vi "APPA207.vi"(4 "error in":T13, 7 "Command":T14) -> (0 "error out":T13, 3 "Response":T11)   [LabVIEW 2018]
uses:
  MOKO_LabViewLibrary/MokoLowLevel/MokoLowLovelControl/MLLC_Command.ctl
  MOKO_LabViewLibrary/MokoLowLevel/MokoLowLovelControl/MLLC_Error.ctl
  MOKO_LabViewLibrary/MokoLowLevel/MokoLowLovelControl/MLLC_Mode.ctl
  MOKO_LabViewLibrary/MokoLowLevel/MokoLowLovelControl/MLLC_Response.ctl
  MOKO_LabViewLibrary/MokoLowLevel/MokoLowLovelControl/MLLC_DriverName.ctl
  MOKO_LabViewLibrary/MokoLowLevel/MokoLowLovelControl/MLLC_Request.ctl
  MOKO_LabViewLibrary/MokoLowLevel/MokoLowLovelControl/MLLC_ErrorCode.ctl
  MOKO_LabViewLibrary/MokoLowLevel/MokoLowLovelControl/MLLC_ConnectCluster.ctl
  MOKO_LabViewLibrary/MokoLowLevel/MokoLowLovelControl/MLLC_InterfaceType.ctl
  MOKO_LabViewLibrary/MokoLowLevel/MokoLowLovelControl/MLLC_OpenedSession.ctl
  MOKO_LabViewLibrary/MokoLowLevel/MokoLowLovelControl/MLLC_InterfaceSettings.ctl
  MOKO_LabViewLibrary/MokoLowLevel/MokoLowLovelControl/MLLC_InterfaceKind.ctl
  MOKO_LabViewLibrary/MokoLowLevel/MokoLowLovelControl/MLLC_ResponseInit.ctl
  MOKO_LabViewLibrary/MokoLowLevel/MokoLowLovelControl/MLLC_Rs232Settings.ctl
panel:
  in  "ResponseInit":T1="OK"
  in  "Settings":T7={"Permanent data"={"Connect"={"InterfaceType"=enum."VISA", "OpenedSession"="", "InterfaceSettings"={"Interface"=enum."RS232", "EOS 4 read"=enum."None", "EOS 4 write"=enum."None", "TMO, ms"=1000, "Sett"=variant(cluster{"Baud Rate":u32, "Data Bits":u16, "Parity":u16, "Stop Bits":u16, "Flow Control":u16, "Eho":bool} {"Baud Rate"=75, "Data Bits"=0, "Parity"=0, "Stop Bits"=0, "Flow Control"=0, "Eho"=FALSE})}}}, "Saved Data"=variant}
  in  "Error Code":T8=5475
  in  "Request":T9="UU\u0000\u0000ª"
  in  "Driver Name":T10="APPA207"
  in  "Mode":T12=enum."Check"
  # "APPA207"
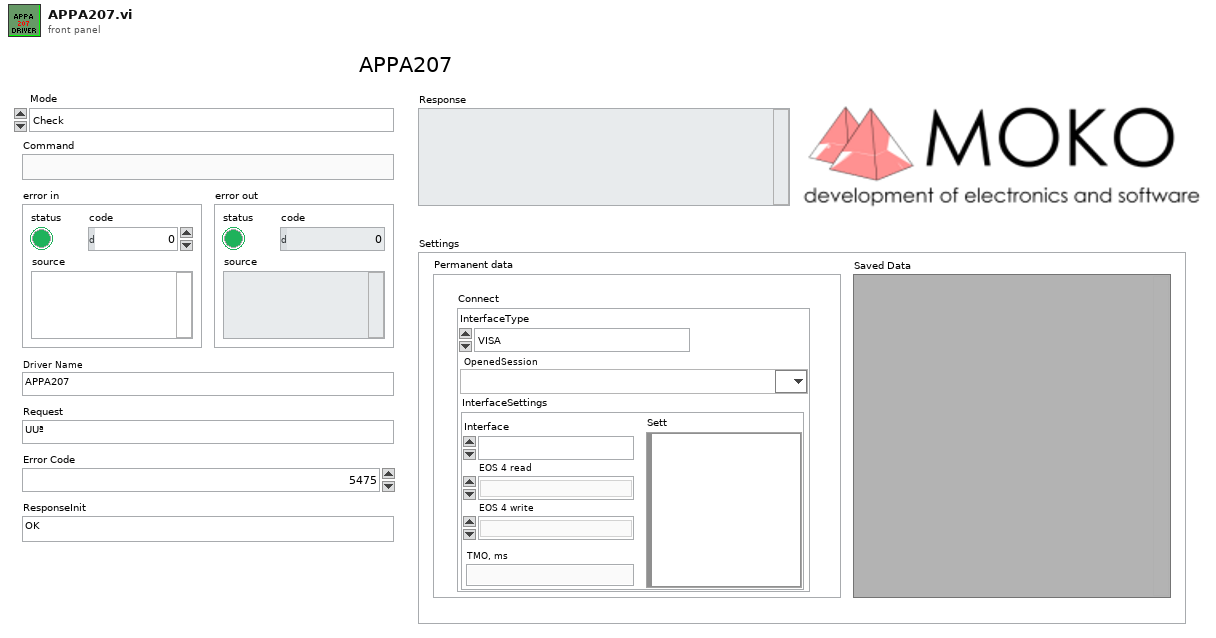
[diagram p1: front panel]
types:
  T1 = typedef "MLLC_ResponseInit.ctl" = string
  T2 = typedef "MLLC_ConnectCluster.ctl" = cluster{"InterfaceType":T3, "OpenedSession":T4, "InterfaceSettings":T5}
  T3 = typedef "MLLC_InterfaceType.ctl" = enum16{"VISA", "Prologix USB-GPIB"}
  T4 = typedef "MLLC_OpenedSession.ctl" = refnum<visa-resource-name>
  T5 = typedef "MLLC_InterfaceSettings.ctl" = cluster{"Interface":T6, "EOS 4 read":enum16{"Default (=EOS 4 write)", "CR (\\r)", "LF (\\n)", "None"}, "EOS 4 write":enum16{"CR+LF (\\r\\n)", "CR (\\r)", "LF (\\n)", "None"}, "TMO, ms":i32, "Sett":variant}
  T6 = typedef "MLLC_InterfaceKind.ctl" = enum16{"RS232", "GPIB", "USB", "Ethernet", "another"}
  T7 = cluster{"Permanent data":cluster{"Connect":T2}, "Saved Data":variant}
  T8 = typedef "MLLC_ErrorCode.ctl" = u32
  T9 = typedef "MLLC_Request.ctl" = string
  T10 = typedef "MLLC_DriverName.ctl" = string
  T11 = typedef "MLLC_Response.ctl" = string
  T12 = typedef "MLLC_Mode.ctl" = enum16{"get", "set", "close", "Init", "Check"}
  T13 = typedef "MLLC_Error.ctl" = errorcluster
  T14 = typedef "MLLC_Command.ctl" = string
  T15 = typedef "MLLC_Rs232Settings.ctl" = cluster{"Baud Rate":u32, "Data Bits":u16, "Parity":u16, "Stop Bits":u16, "Flow Control":u16, "Eho":bool, "Address":dbl}
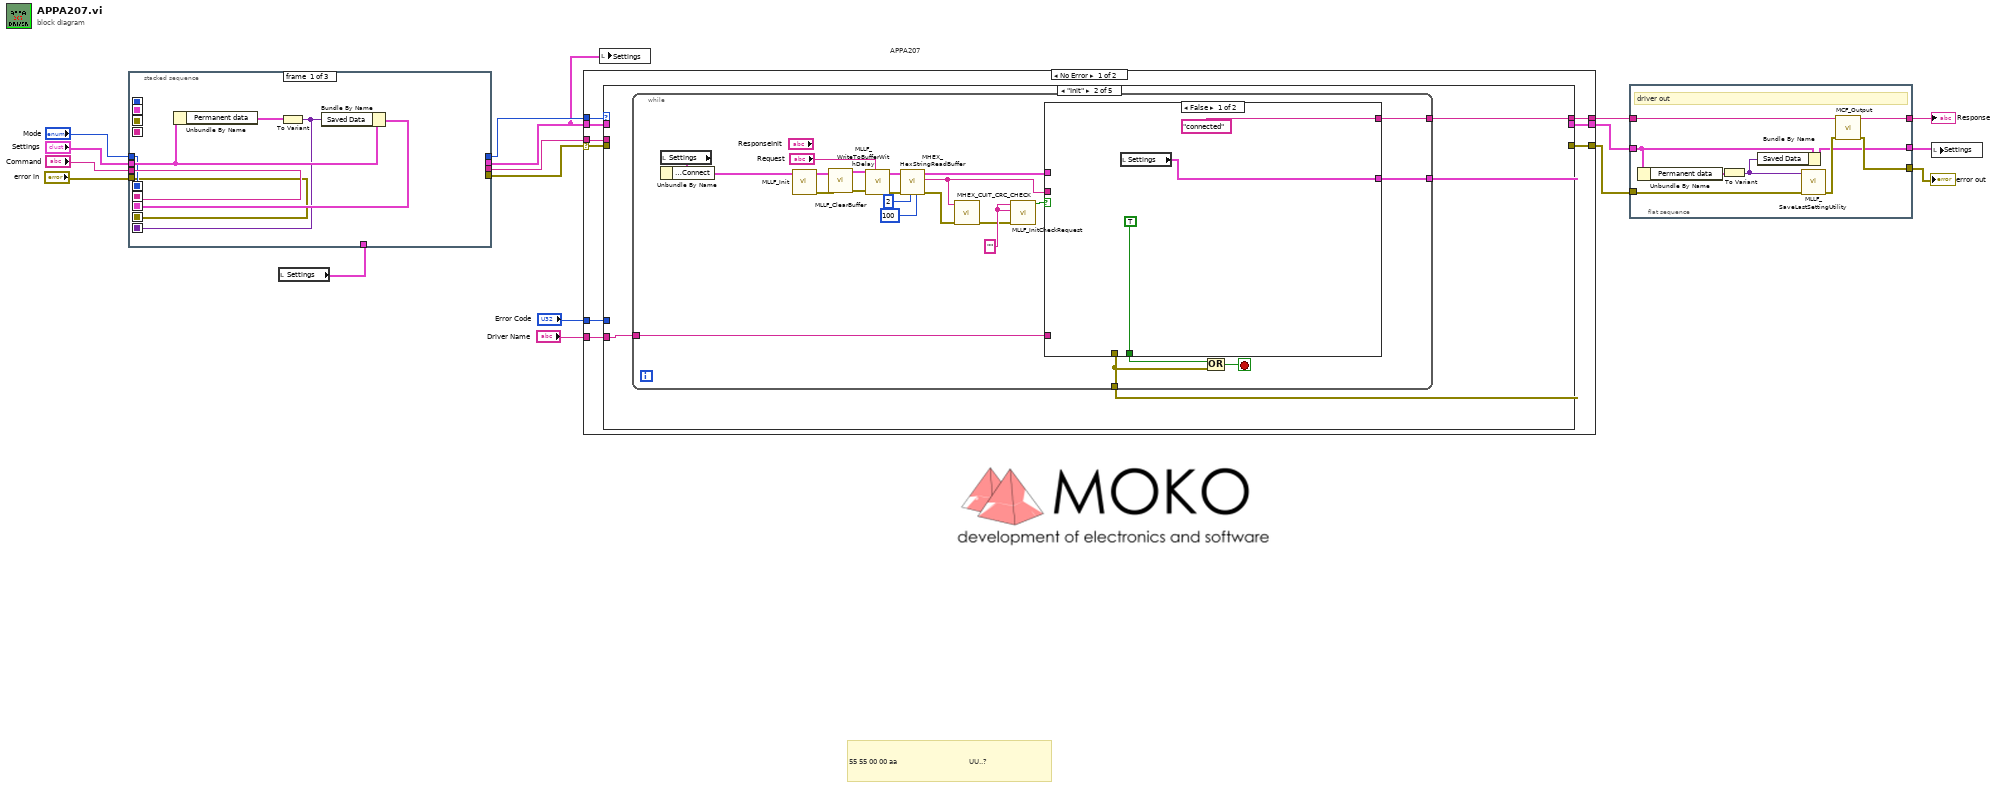
[diagram p0: block diagram]
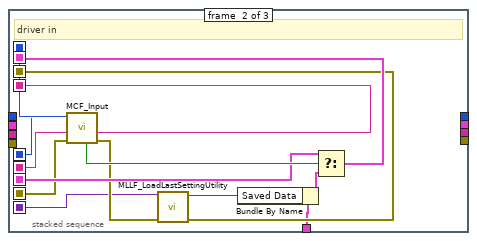
[diagram p2: hidden frame]
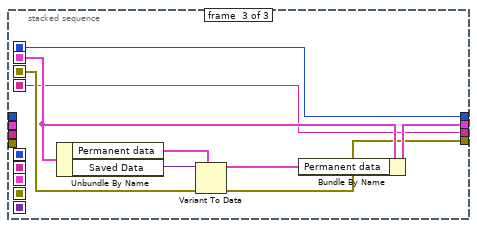
[diagram p3: hidden frame]
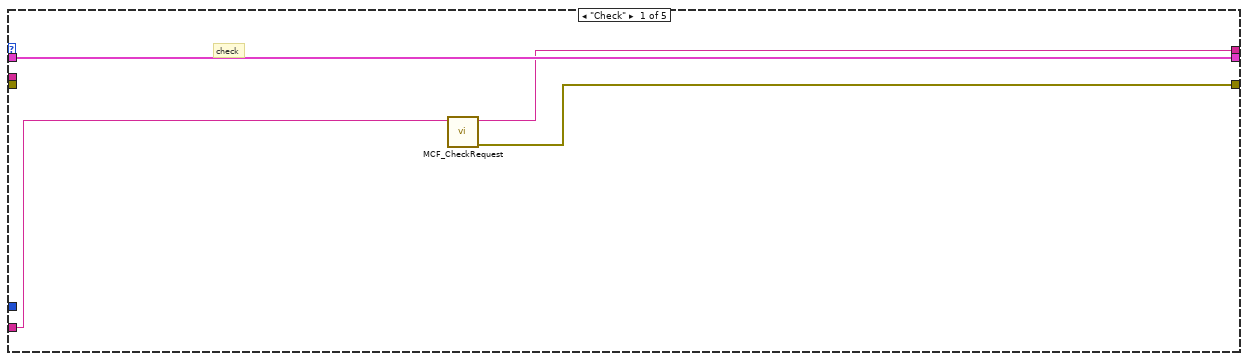
[diagram p4: hidden frame]
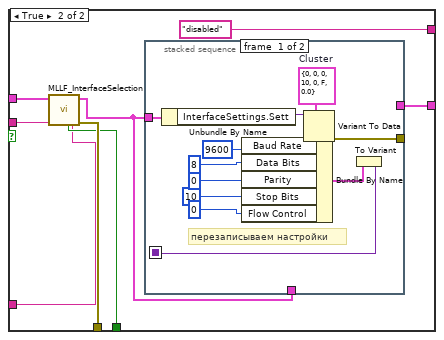
[diagram p5: hidden frame]
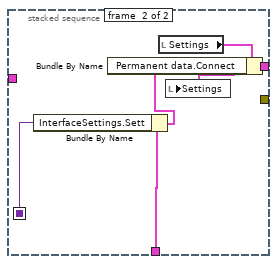
[diagram p6: hidden frame]
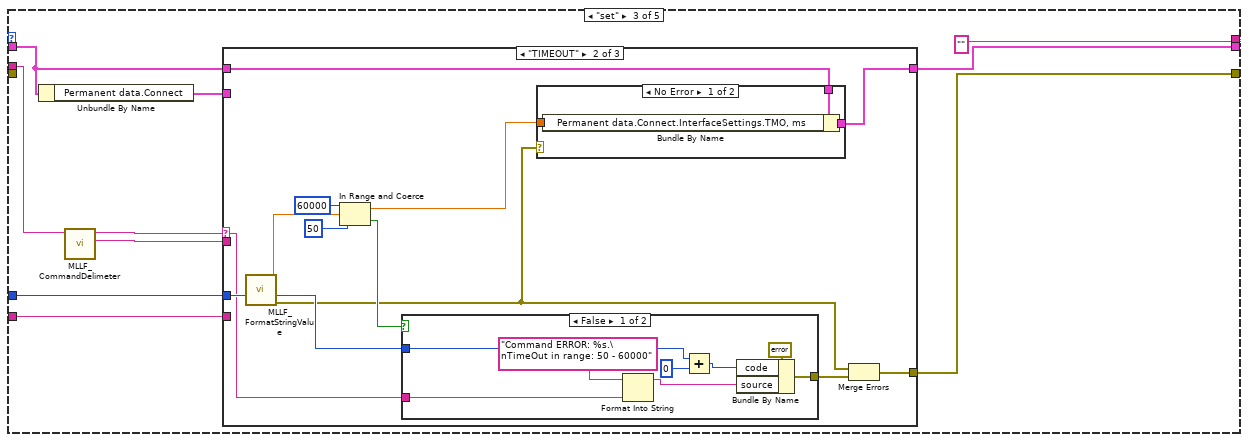
[diagram p7: hidden frame]
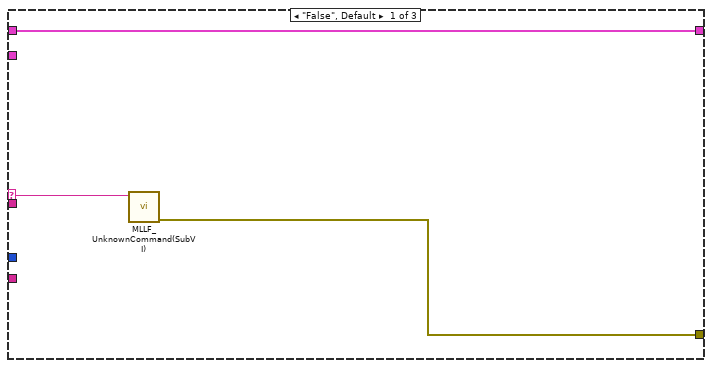
[diagram p8: hidden frame]
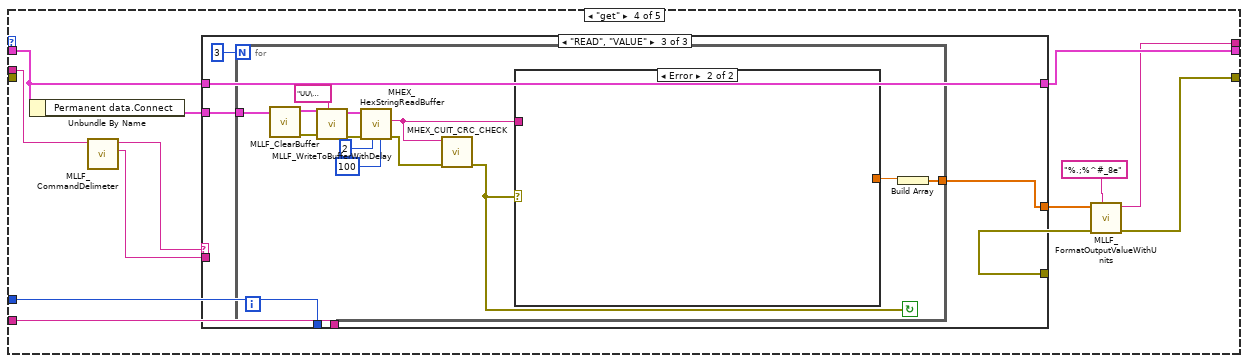
[diagram p12: hidden frame]
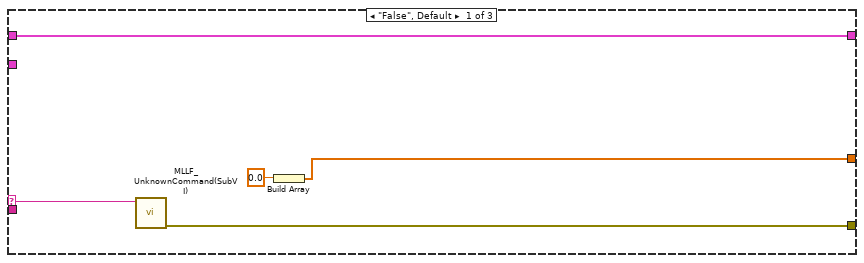
[diagram p13: hidden frame]
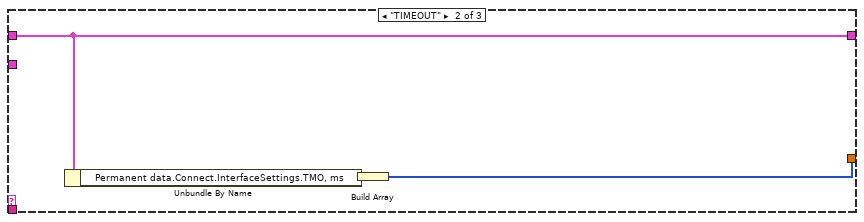
[diagram p14: hidden frame]
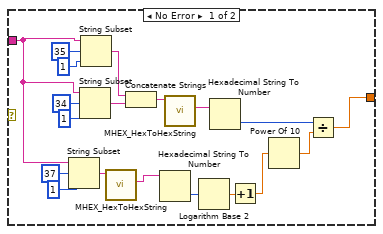
[diagram p15: hidden frame]
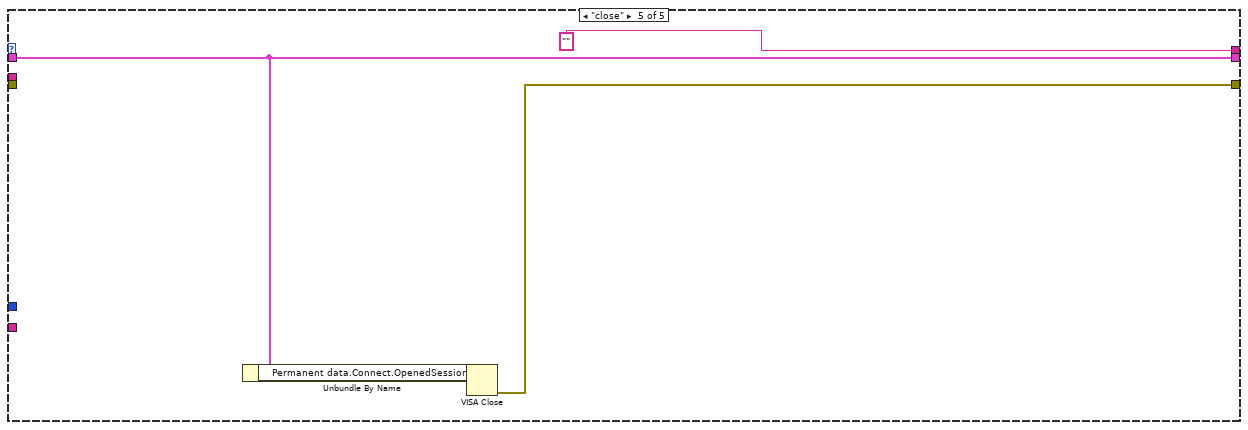
[diagram p16: hidden frame]
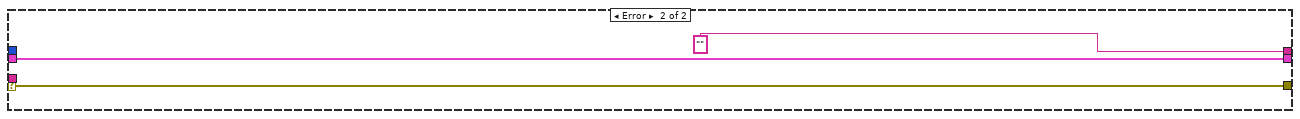
[diagram p17: hidden frame]
diagram:
  # "55 55 00 00 aa                                    UU..?"
  # "APPA207"
  n1 = local read "Settings"() -> (w11:T7)
  n2 = stacked-sequence {
    seq-local: [w20 _ _] -> [_ w36 _]
    seq-local: [w19 _ _] -> [_ w37 _]
    seq-local: [w22 _ _] -> [_ w32 _]
    seq-local: [w18 _ _] -> [_ w31 _]
    seq-local: [w21 _ _] -> [_ w27 _]
    seq-local: [_ w28 _] -> [_ _ w44]
    seq-local: [_ w38 _] -> [_ _ w41]
    seq-local: [_ w35 _] -> [_ _ w40]
    seq-local: [_ w34 _] -> [_ _ w45]
    tunnel: "Command" -> [w20 _ _]
    tunnel: "Mode" -> [w19 _ _]
    tunnel: "error in" -> [w18 _ _]
    tunnel: "Settings" -> [w23 _ _]
    tunnel: w11 -> [_ w26 _]
    tunnel: [_ _ w40] -> w8
    tunnel: [_ _ w43] -> w9
    tunnel: [_ _ w42] -> w7
    tunnel: [_ _ w41] -> w10
    frame #0 {
      n3 = Unbundle By Name(w23) -> ("Permanent data"=w24:cluster{"Connect":T2})
      n4 = To Variant(anything=w24) -> (Variant=w21:variant)
      n5 = Bundle By Name(cluster=w23, "Saved Data"=w21) -> (w22:T7)
    }
    frame #1 {
      # "driver in"
      n6 = call "MCF_Input.vi"("Error In"=w31, "Command in"=w36, "Mode in"=w37) -> ("Error Out"=w30:errorcluster, "Command out"=w35:string, "Mode out"=w38:T12, "Boolean"=w33:bool)  [unwired: 5 in]
      n7 = call "MLLF_LoadLastSettingUtility.vi"("Error In"=w30, "Save data in"=w27) -> ("Error Out"=w28:errorcluster, "Save data out"=w25:variant)  [unwired: 8 in]
      n8 = Bundle By Name(cluster=w26, "Saved Data"=w25) -> (w29:T7)
      n9 = Select(t=w32, s=w33, f=w29) -> (s? t:f=w34:T7)
    }
    frame #2 {
      n10 = Unbundle By Name(w45) -> ("Permanent data"=w46:cluster{"Connect":T2}, "Saved Data"=w39:variant)
      n11 = Variant To Data(error in=w44, type=w46, Variant=w39) -> (data=w47:cluster{"Connect":T2}, error out=w42:errorcluster)
      n12 = Bundle By Name(cluster=w45, "Permanent data"=w47) -> (w43:T7)
    }
  }
  n13 = case shown="No Error" w7 {
    selector: w7 -> [w52 w217]
    tunnel: [w54 w217] -> w4
    tunnel: w10 -> [w56 _]
    tunnel: [w55 "" ("String")] -> w6
    tunnel: w8 -> [w53 _]
    tunnel: w9 -> [w49 w216]
    tunnel: "Error Code" -> [w51 _]
    tunnel: "Driver Name" -> [w50 _]
    tunnel: [w48 w216] -> w5
    frame No Error {
      n14 = case shown="\"Init\"" w56 {
        tunnel: [w58 w64 "" ("String") w159 "" ("String")] -> w55
        tunnel: [w59 w62 w116 w160 w213] -> w54
        tunnel: w53 -> [_ _ w119 w158 _]
        tunnel: w52 -> [_ _ _ _ _]
        tunnel: w51 -> [_ _ w125 w165 _]
        tunnel: w50 -> [w57 w61 w122 w164 _]
        tunnel: w49 -> [w60 _ w124 w155 w212]
        tunnel: [w60 w63 w123 w166 w212] -> w48
        frame "Check" {
          # "check"
          n15 = call "MCF_CheckRequest.vi"("Driver Name"=w57) -> ("Error Out"=w59:errorcluster, "Output String"=w58:string)  [unwired: 9 in]
        }
        frame "Init" {
          n16 = while {
            tunnel: [w83] -> w62
            tunnel: [w81] -> w64
            tunnel: [w80] -> w63
            tunnel: w61 -> [w66]
            stop <- w82 stop-if-true
            w69 = ""
            n17 = local read "Settings"() -> (w87:T7)
            n18 = Unbundle By Name(w87) -> ("Permanent data.Connect"=w85:T2)
            n19 = call "MLLF_Init.vi"("DriverConnect in"=w85) -> ("Error Out"=w74:errorcluster, "DriverConnect out"=w75:T2)  [unwired: 7 in]
            n20 = call "MLLF_ClearBuffer.vi"("Error In"=w74, "DriverConnect in"=w75) -> ("Error Out"=w72:errorcluster, "DriverConnect out"=w73:T2)  [unwired: 6 in, 1 out]
            n21 = call "MLLF_WriteToBufferWithDelay.vi"("Command"="Request", "Error In"=w72, "DriverConnect in"=w73) -> ("Error Out"=w77:errorcluster, "DriverConnect out"=w78:T2)  [unwired: 7 in]
            n22 = call "MHEX_HexStringReadBuffer.vi"("byte count"=u32 100, "length (rest)"=2, "error in"=w77, "DriverConnect in"=w78) -> ("error out"=w67:T13, "String from device out"=w65:string, "DriverConnect out"=w76:T2)  [unwired: 4 in, 1 out]
            n23 = call "MHEX_CUIT_CRC_CHECK.vi"("Error In"=w67, "string in"=w65) -> ("Error Out"=w68:errorcluster)  [unwired: 9 in]
            n24 = call "MLLF_InitCheckRequest.vi"("error in (no error)"=w68, "Answer"=w69, "Response Init"=w69) -> ("Design"=w79:bool)  [unwired: 5 in, 3 out]
            n25 = case shown="False" w79 {
              tunnel: w76 -> [_ w98]
              tunnel: [TRUE w95] -> w84
              tunnel: [_ w97] -> w83
              tunnel: ["connected" "disabled"] -> w81
              tunnel: [w88 w93] -> w80
              tunnel: w66 -> [_ w92]
              tunnel: w65 -> [_ w91]
              frame False {
                n26 = local read "Settings"() -> (w88:T7)
              }
              frame True {
                n27 = call "MLLF_InterfaceSelection.vi"("Driver Name"=w92, "Answer:"=w91, "DriverConnect in"=w98) -> ("error out"=w97:T13, "DriverConnect out"=w94:T2, "stop init?"=w95:bool)  [unwired: 4 in, 2 out]
                n28 = stacked-sequence {
                  seq-local: [w100 _] -> [_ w114]
                  tunnel: w94 -> [w101 _]
                  tunnel: w94 -> [_ w113]
                  tunnel: [_ w111] -> w93
                  tunnel: [w99 _] -> _
                  frame #0 {
                    w104 = T15 {"Baud Rate"=0, "Data Bits"=0, "Parity"=0, "Stop Bits"=10, "Flow Control"=0, "Eho"=FALSE, "Address"=0.0}  # Cluster
                    # "перезаписываем настройки"
                    n29 = Unbundle By Name(w101) -> ("InterfaceSettings.Sett"=w103:variant)
                    n30 = Variant To Data(type=w104, Variant=w103) -> (data=w105:T15, error out=w99:errorcluster)  [unwired: 1 in]
                    n31 = Bundle By Name(cluster=w105, "Baud Rate"=u32 9600, "Data Bits"=u16 8 ("Serial Settings:Data Bits"), "Parity"=u16 0 ("Serial Settings:Parity"), "Stop Bits"=u16 10 ("Serial Settings:Stop Bits"), "Flow Control"=u16 0 ("Serial Settings:Flow Control")) -> (w110:T15)
                    n32 = To Variant(anything=w110) -> (Variant=w100:variant)
                  }
                  frame #1 {
                    n33 = Bundle By Name(cluster=w113, "InterfaceSettings.Sett"=w114) -> (w112:T2)
                    n34 = local read "Settings"() -> (w115:T7)
                    n35 = Bundle By Name(cluster=w115, "Permanent data.Connect"=w112) -> (w111:T7)
                    n36 = local write "Settings"(w111) -> ()
                  }
                }
              }
            }
            n37 = Or(x=w84, y=w83) -> (x .or. y?=w82:bool)
          }
        }
        frame "set" {
          n38 = Unbundle By Name(w124) -> ("Permanent data.Connect"=w120:T2)
          n39 = call "MLLF_CommandDelimeter.vi"("command with param"=w119) -> ("param 1"=w117:string, "command"=w118:string)  [unwired: 6 in, 3 out]
          n40 = case shown="\"TIMEOUT\"" w118 {
            selector: w118 -> [w127 w129 _]
            tunnel: w117 -> [_ _ _]
            tunnel: [w126 w134 _] -> w116
            tunnel: w125 -> [_ w135 _]
            tunnel: w124 -> [w128 w139 w153]
            tunnel: [w128 w140 w153] -> w123
            tunnel: w120 -> [_ _ _]
            tunnel: w122 -> [_ _ _]
            frame "False", Default {
              n41 = call "MLLF_UnknownCommand(SubVI).vi"("Unknown command"=w127) -> ("error out"=w126:errorcluster)  [unwired: 10 in]
            }
            frame "TIMEOUT" {
              n42 = call "MLLF_FormatStringValue.vi"() -> ("error out"=w130:T13, "number"=w131:dbl)  [unwired: 9 in, 1 out]
              n43 = In Range and Coerce(upper limit=60000, x=w131, lower limit=50) -> (coerced(x)=w136:dbl, In Range?=w132:bool)
              n44 = case shown="False" w132 {
                tunnel: [w147 _] -> w133
                tunnel: w135 -> [w146 _]
                tunnel: w129 -> [w145 _]
                frame False {
                  n45 = Format Into String(format string="Command ERROR: %s.\nTimeOut in range: 50 - 60000", w145) -> (resulting string=w149:string)  [unwired: 2 in, 1 out]
                  n46 = Add(x=w146, y=0) -> (x+y=w150:T8)
                  n47 = Bundle By Name(cluster=errorcluster {"status"=TRUE, "code"=0, "source"=""} ("error out"), "code"=w150, "source"=w149) -> (w147:errorcluster)
                }
                frame True {
                }
              }
              n48 = case shown="No Error" w130 {
                tunnel: [w143 w144] -> w140
                tunnel: w139 -> [w142 w144]
                tunnel: w136 -> [w141 _]
                frame No Error {
                  n49 = Bundle By Name(cluster=w142, "Permanent data.Connect.InterfaceSettings.TMO, ms"=w141) -> (w143:T7)
                }
                frame Error {
                }
              }
              n50 = Merge Errors(w130, w133) -> (w134:errorcluster)
            }
            frame "<----MAIN FUNCTIONS---->" {
            }
          }
        }
        frame "get" {
          n51 = Unbundle By Name(w155) -> ("Permanent data.Connect"=w154:T2)
          n52 = call "MLLF_CommandDelimeter.vi"("command with param"=w158) -> ("param 1"=w156:string, "command"=w157:string)  [unwired: 6 in, 3 out]
          n53 = case shown="\"READ\", \"VALUE\"" w157 {
            selector: w157 -> [w168 _ _]
            tunnel: [w167 _ _] -> w163
            tunnel: w165 -> [_ _ _]
            tunnel: [w171 w174 w177] -> w166
            tunnel: w155 -> [w171 w174 w177]
            tunnel: [w169 w172 w175] -> w162
            tunnel: w164 -> [_ _ _]
            tunnel: w156 -> [_ _ _]
            tunnel: w154 -> [_ _ w178]
            frame "False", Default {
              n54 = call "MLLF_UnknownCommand(SubVI).vi"("Unknown command"=w168) -> ("error out"=w167:errorcluster)  [unwired: 10 in]
              n55 = Build Array(0.0 ("TimeOut")) -> (w169:dbl[])
            }
            frame "TIMEOUT" {
              n56 = Unbundle By Name(w174) -> ("Permanent data.Connect.InterfaceSettings.TMO, ms"=w173:i32)
              n57 = Build Array(w173) -> (w172:i32[])
            }
            frame "READ", "VALUE" {
              n58 = for {
                N: 3 -> [_]
                tunnel: w178 -> [w184]
                tunnel: [w179] -> w175
                stop <- w181 continue-if-true
                n59 = call "MLLF_ClearBuffer.vi"("DriverConnect in"=w184) -> ("Error Out"=w187:errorcluster, "DriverConnect out"=w188:T2)  [unwired: 7 in, 1 out]
                n60 = call "MLLF_WriteToBufferWithDelay.vi"("Command"=T9 "UU\u0000\u0000ª" ("Request 2"), "Error In"=w187, "DriverConnect in"=w188) -> ("Error Out"=w189:errorcluster, "DriverConnect out"=w190:T2)  [unwired: 7 in]
                n61 = call "MHEX_HexStringReadBuffer.vi"("byte count"=u32 100, "length (rest)"=2, "error in"=w189, "DriverConnect in"=w190) -> ("error out"=w182:T13, "String from device out"=w183:string)  [unwired: 4 in, 2 out]
                n62 = call "MHEX_CUIT_CRC_CHECK.vi"("Error In"=w182, "string in"=w183) -> ("Error Out"=w181:errorcluster)  [unwired: 9 in]
                n63 = case shown="Error" w181 {
                  tunnel: w183 -> [w204 _]
                  tunnel: [w192 _] -> w180
                  frame No Error {
                    n64 = String Subset(string=w204, offset (0)=37, length (rest)=1 ("length (rest)")) -> (substring=w199:string)
                    n65 = String Subset(string=w204, offset (0)=34, length (rest)=1 ("length (rest)")) -> (substring=w202:string)
                    n66 = String Subset(string=w204, offset (0)=35, length (rest)=1 ("length (rest)")) -> (substring=w203:string)
                    n67 = call "MHEX_HexToHexString.vi"("STRING HEX"=w199) -> ("Without space"=w198:string)  [unwired: 8 in, 2 out]
                    n68 = Concatenate Strings(w203, w202) -> (w201:string)
                    n69 = Hexadecimal String To Number(string=w198) -> (number=w197:u32)  [unwired: 2 in, 1 out]
                    n70 = call "MHEX_HexToHexString.vi"("STRING HEX"=w201) -> ("Without space"=w200:string)  [unwired: 8 in, 2 out]
                    n71 = Logarithm Base 2(1:w197) -> (0:w196:dbl)
                    n72 = Hexadecimal String To Number(string=w200) -> (number=w194:u32)  [unwired: 2 in, 1 out]
                    n73 = Increment(x=w196) -> (x+1=w195:dbl)
                    n74 = Power Of 10(x=w195) -> (10^x=w193:dbl)
                    n75 = Divide(x=w194, y=w193) -> (x/y=w192:dbl)
                  }
                  frame Error {
                  }
                }
                n76 = Build Array(w180) -> (w179:dbl[])
              }
            }
          }
          n77 = call "MLLF_FormatOutputValueWithUnits.vi"("Format"="%.;%^#_8e" ("format string"), "error in"=w163, "ValuesIn"=w162) -> ("error out"=w160:T13, "Result string"=w159:T14)  [unwired: 7 in]
        }
        frame "close" {
          n78 = Unbundle By Name(w212) -> ("Permanent data.Connect.OpenedSession"=w214:T4)
          n79 = VISA Close(VISA resource name=w214) -> (error out=w213:errorcluster)  [unwired: 1 in]
        }
      }
    }
    frame Error {
    }
  }
  n80 = local write "Settings"(w9) -> ()
  n81 = flat-sequence {
    tunnel: [w226] -> w1
    tunnel: [w225] -> w3
    tunnel: w6 -> [w224]
    tunnel: w4 -> [w223]
    tunnel: w5 -> [w219]
    tunnel: [w221] -> w2
    frame #0 {
      # "driver out"
      n82 = Unbundle By Name(w219) -> ("Permanent data"=w218:cluster{"Connect":T2})
      n83 = To Variant(anything=w218) -> (Variant=w220:variant)
      n84 = Bundle By Name(cluster=w219, "Saved Data"=w220) -> (w221:T7)
      n85 = call "MLLF_SaveLastSettingUtility.vi"("error in"=w223, "Saved Data"=w220) -> ("error out"=w222:T13)  [unwired: 8 in, 1 out]
      n86 = call "MCF_Output.vi"("Error In"=w222, "Input"=w224) -> ("Error Out"=w225:errorcluster, "Output"=w226:string)  [unwired: 8 in]
    }
  }
  n87 = local write "Settings"(w2) -> ()
  "error out" <- w3
  "Response" <- w1
